vi "WriteConfigFile.vi"(0 "reference in":refnum<class "DAQ_Base.lvclass">, 1 "ConfigFlieName":string="DAQSetting.ini", 2 "DAQSettings":T1={"SampleSettings"={"samples per channel"=100, "SampleRate"=1000.0, "TansMaxLength"=500000.0, "ReadTimeOut"=10.0, "时钟源"=""}, "AI_ChannelSettings"={"AI_SettingsArry"=[{"DeviceName"="SimDev1", "physical channels"="Dev1/ai0", "AssignName"="输入轴扭矩", "输入信号类型"=10106, "Max_value"=10.0, "Min_value"=-10.0, "单位"=10348, "shunt resistor location"=-1, "external shunt resistor value"=2.0, "标定系数"={"Scale"=0.0, "Offset"=0.0}}, {"DeviceName"="SimDev1", "physical channels"="Dev1/ai1", "AssignName"="输出轴扭矩", "输入信号类型"=10106, "Max_value"=10.0, "Min_value"=-10.0, "单位"=10348, "shunt resistor location"=-1, "external shunt resistor value"=2.0, "标定系数"={"Scale"=0.0, "Offset"=0.0}}]}, "AO_ChannelSettings"={"布尔"=FALSE}, "Cnt_ChannelSettings"={"Cnt_ChannelSettings"=[{"类型"=enum."Linear", "CounterNbr"="SimDev1/ctr0", "AssignName"="输入轴角度", "单位"=10146, "decoding type"=10313, "PPR_DistancePerPulse"=9000.0, "Initial Position "=0.0, "z index enable"=FALSE, "z index phase"=10042, "source"="/SimDev1/ai/SampleClock"}, {"类型"=enum."Rotate", "CounterNbr"="SimDev1/ctr1", "AssignName"="齿条位移", "单位"=10146, "decoding type"=10092, "PPR_DistancePerPulse"=9000.0, "Initial Position "=0.0, "z index enable"=FALSE, "z index phase"=10042, "source"="/SimDev1/ai/SampleClock"}]}} {"Cnt_ChannelSettings"."Cnt_ChannelSettings"."decoding type" items=["X1"=10090, "X2"=10091, "X4"=10092, "双脉冲计数"=10313]; "Cnt_ChannelSettings"."Cnt_ChannelSettings"."z index phase" items=["A High B High"=10040, "A High B Low"=10041, "A Low B High"=10042, "A Low B Low"=10043, ""=0]; "Cnt_ChannelSettings"."Cnt_ChannelSettings"."单位" items=["Radians"=10273, "Degrees"=10146, "Meters"=10219, "Inches"=10379, "Ticks"=10304, "From Custom Scale"=10065]; "AI_ChannelSettings"."AI_SettingsArry"."标定系数"."Offset" format="%_4g"; "AI_ChannelSettings"."AI_SettingsArry"."标定系数"."Scale" format="%.4g"; "AI_ChannelSettings"."AI_SettingsArry"."shunt resistor location" items=["默认"=-1, "内部"=10200, "外部"=10167]; "AI_ChannelSettings"."AI_SettingsArry"."external shunt resistor value" format="%0.2f"; "AI_ChannelSettings"."AI_SettingsArry"."输入信号类型" items=["默认"=-1, "RSE"=10083, "NRSE"=10078, "差分"=10106, "伪差分"=12529]; "AI_ChannelSettings"."AI_SettingsArry"."单位" items=["安培"=10342, "伏特"=10348, "来自自定义换算"=10065]}, 5 "error in (no error)":errorcluster) -> (14 "reference out":refnum<class "DAQ_Base.lvclass">, 19 "error out":errorcluster)   [LabVIEW 2020, in "DAQ.lvlib" / "DAQ_Base.lvclass"]
uses:
  DAQ_Base.lvclass
  protected/DAQSettings.ctl
  protected/SampleSettings.ctl
  protected/AI_ChannelSettings.ctl
  protected/AO_ChannelSettings.ctl
  protected/Cnt_ChannelSettings.ctl
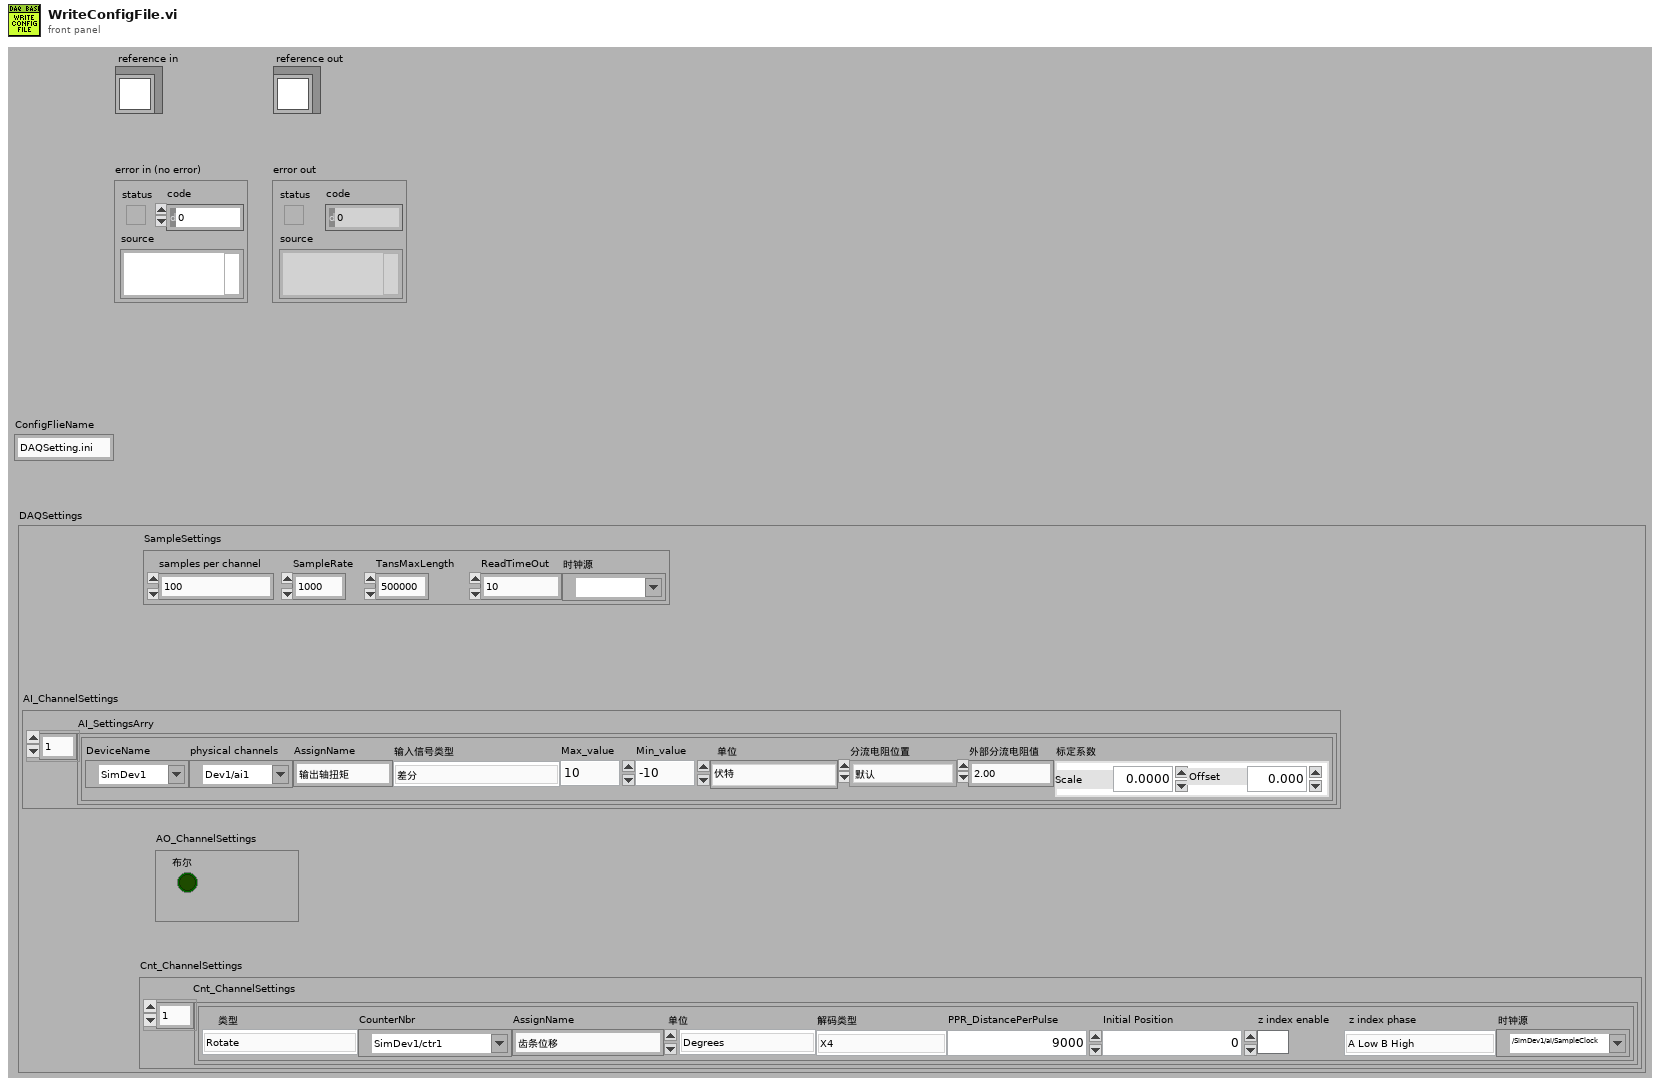
[diagram p1: front panel]
types:
  T1 = typedef "DAQ.lvlib/DAQ_Base.lvclass/DAQSettings.ctl" = cluster{"SampleSettings":T2, "AI_ChannelSettings":T3, "AO_ChannelSettings":T5, "Cnt_ChannelSettings":T6}
  T2 = typedef "DAQ.lvlib/DAQ_Base.lvclass/SampleSettings.ctl" = cluster{"samples per channel":i32, "SampleRate":dbl, "TansMaxLength":dbl, "ReadTimeOut":dbl, "时钟源":tag}
  T3 = typedef "DAQ.lvlib/DAQ_Base.lvclass/AI_ChannelSettings.ctl" = cluster{"AI_SettingsArry":cluster{"DeviceName":tag, "physical channels":tag, "AssignName":string, "输入信号类型":T4, "Max_value":dbl, "Min_value":dbl, "单位":i32, "shunt resistor location":i32, "external shunt resistor value":dbl, "标定系数":cluster{"Scale":dbl, "Offset":dbl}}[]}
  T4 = typedef "AI信号类型.ctl" = i32
  T5 = typedef "DAQ.lvlib/DAQ_Base.lvclass/AO_ChannelSettings.ctl" = cluster{"布尔":bool}
  T6 = typedef "DAQ.lvlib/DAQ_Base.lvclass/Cnt_ChannelSettings.ctl" = cluster{"Cnt_ChannelSettings":cluster{"类型":enum16{"Linear", "Rotate"}, "CounterNbr":tag, "AssignName":string, "单位":u16, "decoding type":u16, "PPR_DistancePerPulse":dbl, "Initial Position ":dbl, "z index enable":bool, "z index phase":i32, "source":tag}[]}
  T7 = typedef "DAQ.lvlib/DAQ_Base.lvclass/ObjectAttributesRef.ctl" = refnum<data-value>
  T8 = typedef "DAQ.lvlib/DAQ_Base.lvclass/ObjectAttributes.ctl" = cluster{"MyAttribute":dbl, "RootPath":path, "DAQSettings":T1, "DaqCollector":cluster{"CollectDataQueue":refnum<queue>, "ArryDataCollectorChannel":T9[], "RealTimeValues":dbl[]}, "CollectorChannelEnable":bool[]}
  T9 = typedef "DAQ.lvlib/DAQ_Base.lvclass/DataCollector.ctl" = cluster{"DataCollectArry":dbl[][], "Update":bool}
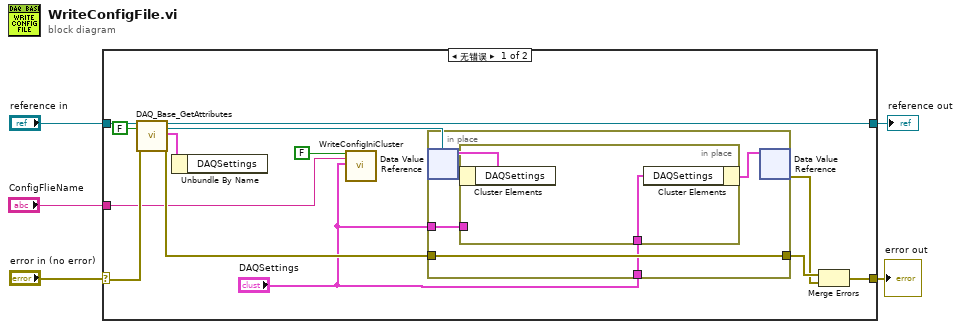
[diagram p0: block diagram]
diagram:
  n1 = case shown="无错误" "error in (no error)" {
    selector: "error in (no error)" -> [w15 w26]
    tunnel: [w18 w26] -> w4
    tunnel: [w16 w25] -> w2
    tunnel: "reference in" -> [w17 w25]
    tunnel: "ConfigFlieName" -> [w8 _]
    frame No Error {
      n2 = call "DAQ_Base_GetAttributes.vi"("reference in"=w17, "return data? (T)"=FALSE, "error in (no error)"=w15) -> ("reference out"=w16:refnum<class "DAQ_Base.lvclass">, "attributes ref"=w10:T7, "attributes"=w13:T8, "error out"=w14:errorcluster)  [unwired: 13 in]
      n3 = Unbundle By Name(w13) -> ()  [unwired: 1 out]
      n4 = call "WriteConfigIniCluster.vi"("更随产品型号变更？"=FALSE, "ConfigFlieName"=w8, "ConfigIn"="DAQSettings") -> ()  [unwired: 16 in, 1 out]
      n5 = in-place {
        in-place-border: w14 -> [w21]
        in-place-border: [w21] -> w12
        in-place-border: "DAQSettings" -> [w20]
        in-place-border: "DAQSettings" -> [w19]
        n6 = in-place-dvr #1(w10) -> (w22:T8)  [unwired: 1 out]
        n7 = in-place {
          in-place-border: w20 -> [_]
          in-place-border: w19 -> [w24]
          n8 = in-place-cluster #2(w22) -> ()  [unwired: 1 out]
          n9 = in-place-cluster #2("DAQSettings"=w24) -> (w23:T8)
        }
        n10 = in-place-dvr #1(w23) -> (w11:errorcluster)  [unwired: 1 out]
      }
      n11 = Merge Errors(w12, w11) -> (w18:errorcluster)
    }
    frame Error {
    }
  }
  "error out" <- w4
  "reference out" <- w2
